vi "toml_value_string.vi"(5 "operation":T1, 6 "modifiers":u16 format="%016b", 7 "section":string[](array[string]), 8 "error in (no error)":errorcluster, 9 "value in":string, 10 "key":string[](array[string]), 11 "path in":path) -> (0 "error out":errorcluster, 1 "value out":string, 2 "exists?":bool, 3 "path out":path)   [LabVIEW 2017]
uses:
  toml_value_operation.ctl
  toml_fg_action.ctl
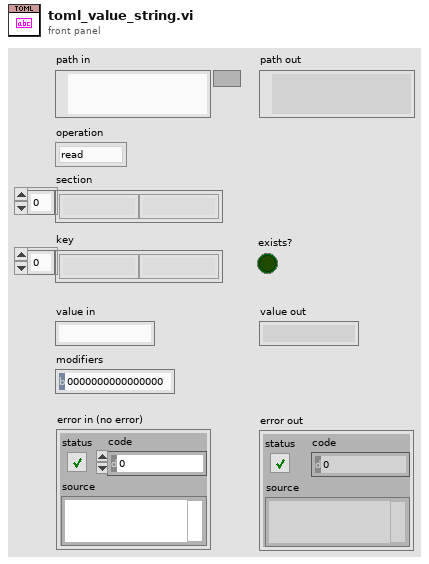
[diagram p1: front panel]
types:
  T1 = typedef "toml_value_operation.ctl" = enum8{"read", "write"}
  T2 = typedef "toml_fg_action.ctl" = enum8{"null", "get", "set", "pop", "import", "export", "drop", "sections", "keys", "remove"}
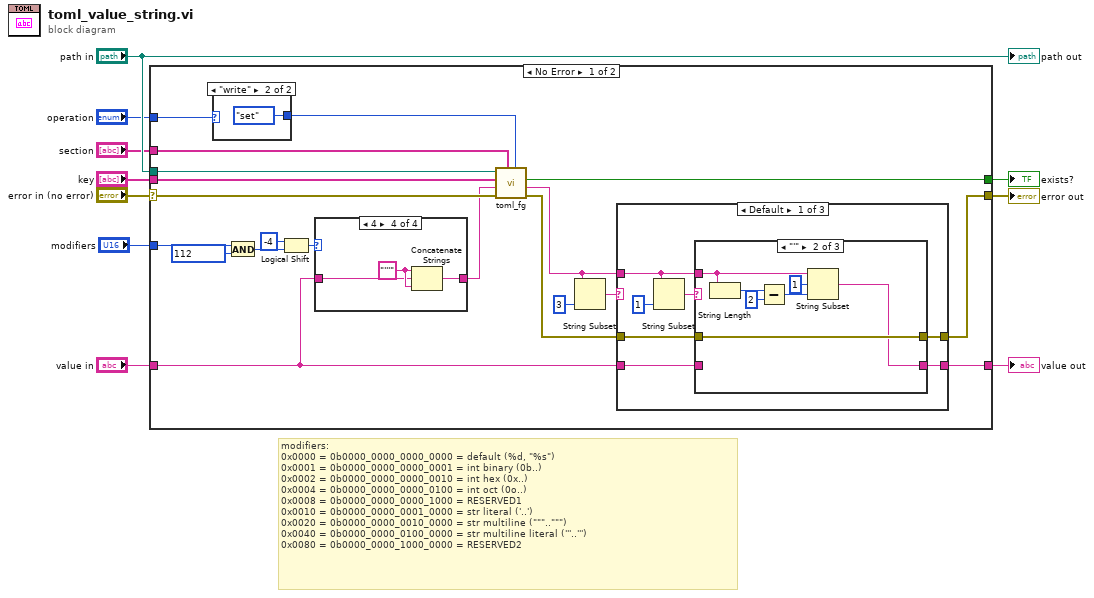
[diagram p0: block diagram]
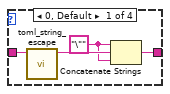
[diagram p2: hidden frame]
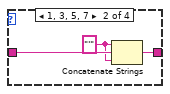
[diagram p3: hidden frame]
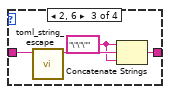
[diagram p4: hidden frame]
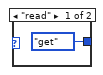
[diagram p5: hidden frame]
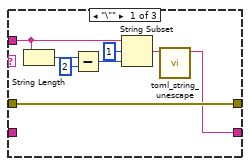
[diagram p6: hidden frame]
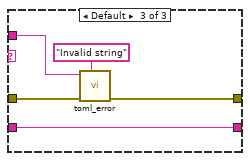
[diagram p7: hidden frame]
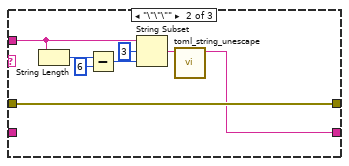
[diagram p8: hidden frame]
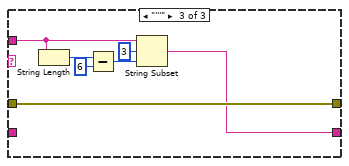
[diagram p9: hidden frame]
diagram:
  # "modifiers:\n0x0000 = 0b0000_0000_0000_0000 = default (%d, \"%s\")\n0x0001 = 0b0000_0000_0000_0001 = int binary (0b..)\n0x0002 = 0b0000_0000_0000_0010 = int hex (0x..)\n0x0004 = 0b0000_0000_0000_0100 = int oct (0o..)\n0x0008 = 0b0000_0000_0000_1000 = RESERVED1\n0x0010 = 0b0000_0000_0001_0000 = str literal ('..')\n0x0020 = 0b0000_0000_0010_0000 = str multiline (\"\"\"..\"\"\")\n0x0040 = 0b0000_0000_0100_0000 = str multiline literal ('''..''')\n0x0080 = 0b0000_0000_1000_0000 = RESERVED2"
  n1 = case shown="No Error" "error in (no error)" {
    selector: "error in (no error)" -> [w30 w90]
    tunnel: [w21 w90] -> w9
    tunnel: "path in" -> [w29 _]
    tunnel: "operation" -> [w27 _]
    tunnel: "section" -> [w26 _]
    tunnel: "key" -> [w25 _]
    tunnel: [w24 _] -> w4
    tunnel: [w23 w89] -> w3
    tunnel: "value in" -> [w11 w89]
    tunnel: "modifiers" -> [w18 _]
    frame No Error {
      n2 = case shown="\"write\"" w27 {
        tunnel: [toml_fg_action."get" ("action") toml_fg_action."set" ("action")] -> w28
        frame "read" {
        }
        frame "write" {
        }
      }
      n3 = And(x=w18, y=u16 112) -> (x .and. y?=w16:u16)
      n4 = Logical Shift(y=i16 -4, x=w16) -> (x << y=w12:u16)
      n5 = case shown="4" w12 {
        tunnel: w11 -> [w34 w37 w40 w42]
        tunnel: [w32 w36 w39 w43] -> w13
        frame 0, Default {
          w31 = "\"" ("string")
          n6 = call "toml_string_escape.vi"("string"=w34) -> ("escaped string"=w33:string)  [unwired: 10 in]
          n7 = Concatenate Strings(w31, w33, w31) -> (w32:string)
        }
        frame 1, 3, 5, 7 {
          w35 = "'" ("string")
          n8 = Concatenate Strings(w35, w37, w35) -> (w36:string)
        }
        frame 2, 6 {
          w38 = "\"\"\"" ("string")
          n9 = call "toml_string_escape.vi"("string"=w40) -> ("escaped string"=w41:string)  [unwired: 10 in]
          n10 = Concatenate Strings(w38, w41, w38) -> (w39:string)
        }
        frame 4 {
          w44 = "'''" ("string")
          n11 = Concatenate Strings(w44, w42, w44) -> (w43:string)
        }
      }
      n12 = call "toml_fg.vi"("action"=w28, "section"=w26, "error in (no error)"=w30, "value in"=w13, "key"=w25, "path in"=w29) -> ("error out"=w22:errorcluster, "value out"=w14:string, "exists?"=w24:bool)  [unwired: 2 in, 1 out]
      n13 = String Subset(string=w14, length (rest)=3 ("length (rest)")) -> (substring=w19:string)  [unwired: 1 in]
      n14 = case shown="Default" w19 {
        tunnel: [w48 w74 w82] -> w23
        tunnel: [w52 w81 w88] -> w21
        tunnel: w22 -> [w53 w81 w88]
        tunnel: w11 -> [w47 _ _]
        tunnel: w14 -> [w50 w80 w87]
        frame Default {
          n15 = String Subset(string=w50, length (rest)=1 ("length (rest)")) -> (substring=w49:string)  [unwired: 1 in]
          n16 = case shown="\"'\"" w49 {
            tunnel: w53 -> [w61 w68 w73]
            tunnel: [w61 w68 w72] -> w52
            tunnel: w50 -> [w55 w63 w70]
            tunnel: [w54 w62 w69] -> w48
            tunnel: w47 -> [_ _ w69]
            frame "\"" {
              n17 = String Length(string=w55) -> (length=w59:i32)
              n18 = Subtract(x=w59, y=2 ("x")) -> (x-y=w58:i32)
              n19 = String Subset(string=w55, offset (0)=1, length (rest)=w58) -> (substring=w56:string)
              n20 = call "toml_string_unescape.vi"("escaped string"=w56) -> ("string out"=w54:string)  [unwired: 9 in, 1 out]
            }
            frame "'" {
              n21 = String Length(string=w63) -> (length=w66:i32)
              n22 = Subtract(x=w66, y=2 ("x")) -> (x-y=w65:i32)
              n23 = String Subset(string=w63, offset (0)=1, length (rest)=w65) -> (substring=w62:string)
            }
            frame Default {
              n24 = call "toml_error.vi"("message"="Invalid string", "error in (no error)"=w73, "toml"=w70) -> ("error out"=w72:errorcluster)  [unwired: 8 in]
            }
          }
        }
        frame "\"\"\"" {
          n25 = String Length(string=w80) -> (length=w78:i32)
          n26 = Subtract(x=w78, y=6 ("x")) -> (x-y=w77:i32)
          n27 = String Subset(string=w80, offset (0)=3, length (rest)=w77) -> (substring=w75:string)
          n28 = call "toml_string_unescape.vi"("escaped string"=w75) -> ("string out"=w74:string)  [unwired: 9 in, 1 out]
        }
        frame "'''" {
          n29 = String Length(string=w87) -> (length=w85:i32)
          n30 = Subtract(x=w85, y=6 ("x")) -> (x-y=w84:i32)
          n31 = String Subset(string=w87, offset (0)=3, length (rest)=w84) -> (substring=w82:string)
        }
      }
    }
    frame Error {
    }
  }
  "error out" <- w9
  "value out" <- w3
  "exists?" <- w4
  "path out" <- "path in"
